vi "MotorOnOff.vi"(7 "#Axis":i32, 8 "error in":errorcluster, 10 "Enabled":bool, 11 "VISA resource":refnum<visa-resource-name>) -> (0 "error out":errorcluster)   [LabVIEW 2012, in "Micos_uic.lvlib"]
uses:
  Micos_uic.lvlib
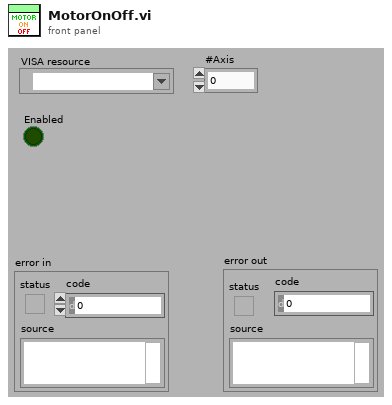
[diagram p1: front panel]
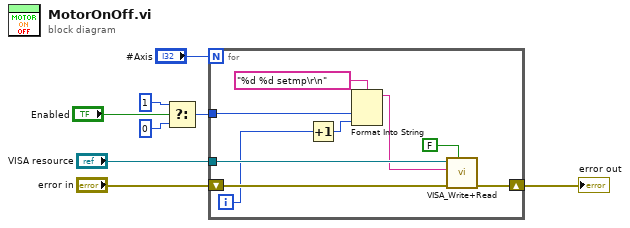
[diagram p0: block diagram]
diagram:
  n1 = Select(t=i8 1, s="Enabled", f=i8 0) -> (s? t:f=w4:i8)
  n2 = for {
    N: "#Axis" -> [_]
    tunnel: "VISA resource" -> [w17]
    tunnel: w4 -> [w14]
    shift-right: [w15] -> w6
    shift-left: "error in" -> [w16]
    i -> [w10]
    n3 = Increment(x=w10) -> (x+1=w11:i32)
    n4 = Format Into String(format string="%d %d setmp\r\n", w14, w11) -> (resulting string=w9:string)  [unwired: 2 in, 1 out]
    n5 = call "VISA_Write+Read.vi"("Read?"=FALSE, "error in (no error)"=w16, "Write Buffer"=w9, "VISA resource name"=w17) -> ("error out"=w15:errorcluster)  [unwired: 5 in, 2 out]
  }
  "error out" <- w6
